vi "fu_gesamt.vi"(8 "Boolean":bool) -> (0 "Frequenz":dbl, 1 "Drehmoment":dbl format="%.2f", 2 "Leistung":dbl, 3 "Drehzahl":dbl, 11 "Scaled":dbl[](array[numeric]) format="%.2f")   [LabVIEW 2015]
uses:
  <vilib>/Instr/_visa.llb/VISA Configure Serial Port (Instr).vi
panel:
  out "return count":u32
  out "subarray":i8[](array[numeric])
  out "read buffer":string
  in  "VISA Refnum in":refnum<visa-resource-name>="COM1"
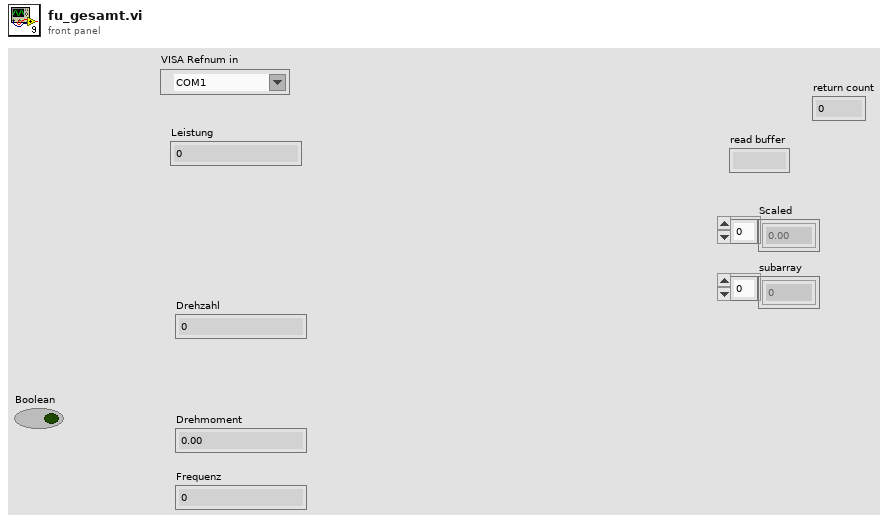
[diagram p1: front panel]
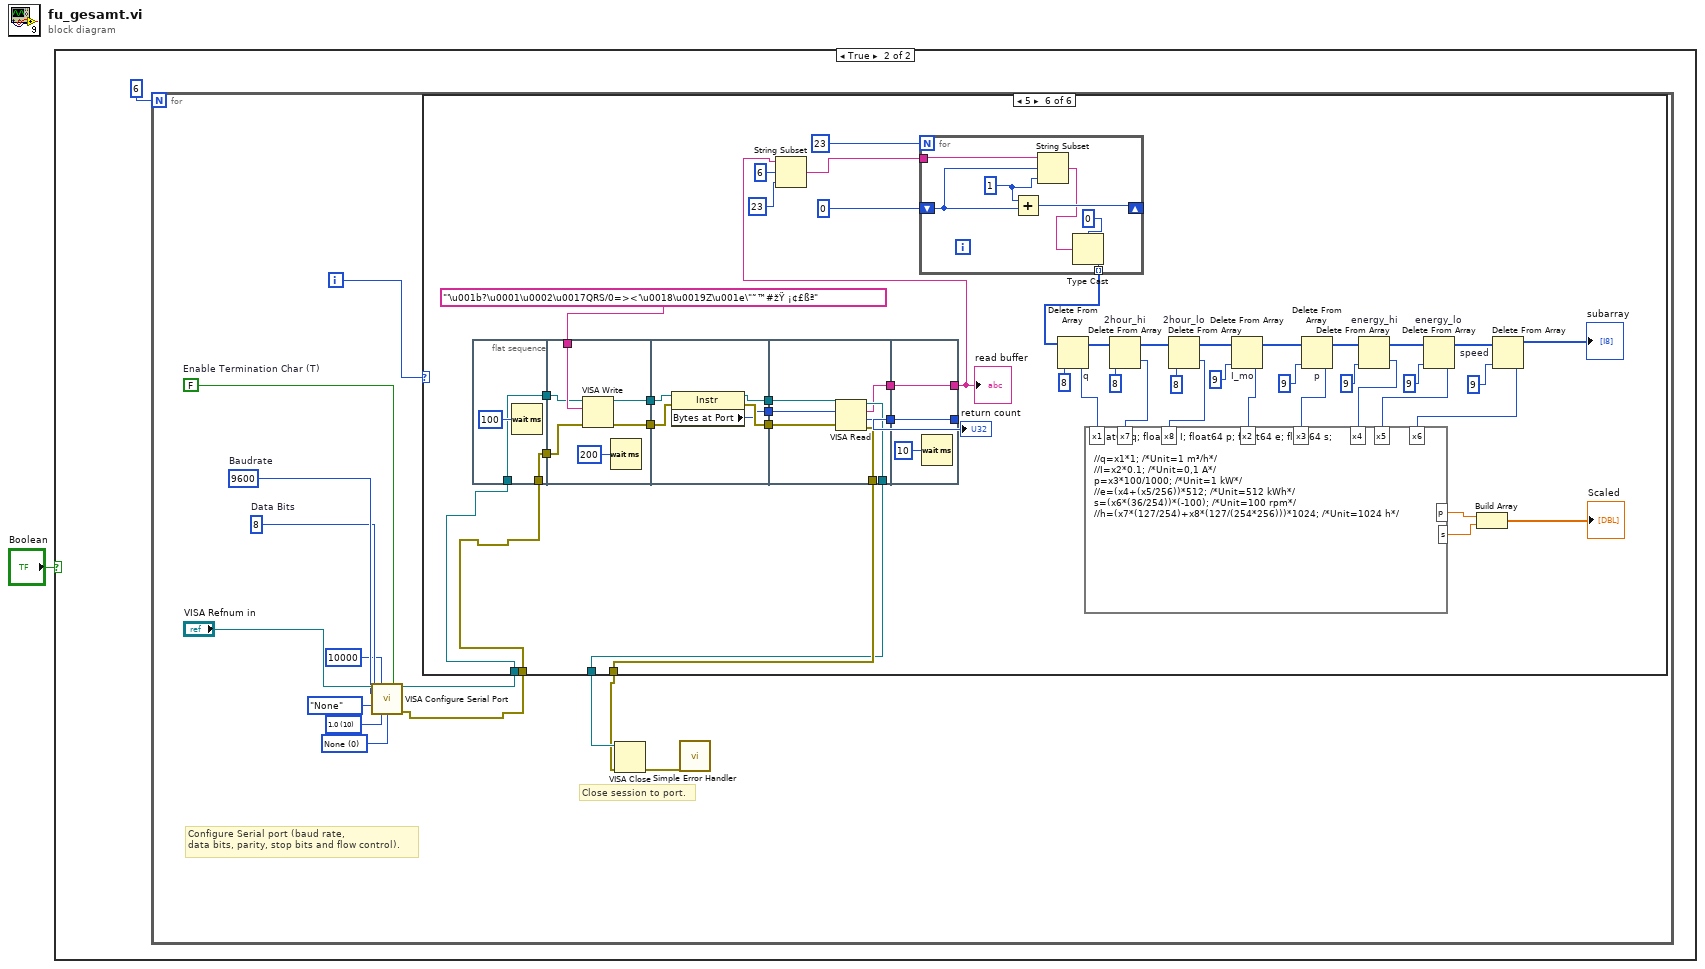
[diagram p0: block diagram]
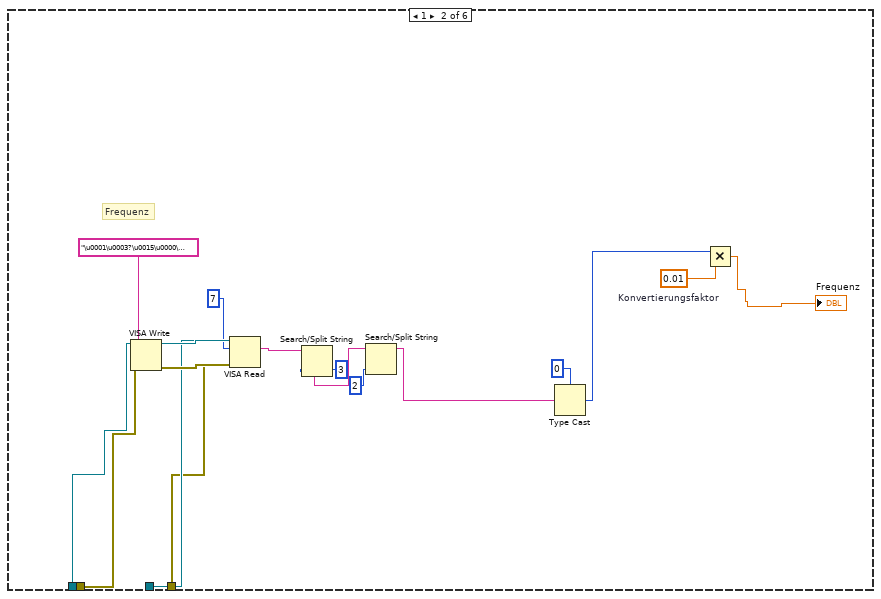
[diagram p4: hidden frame]
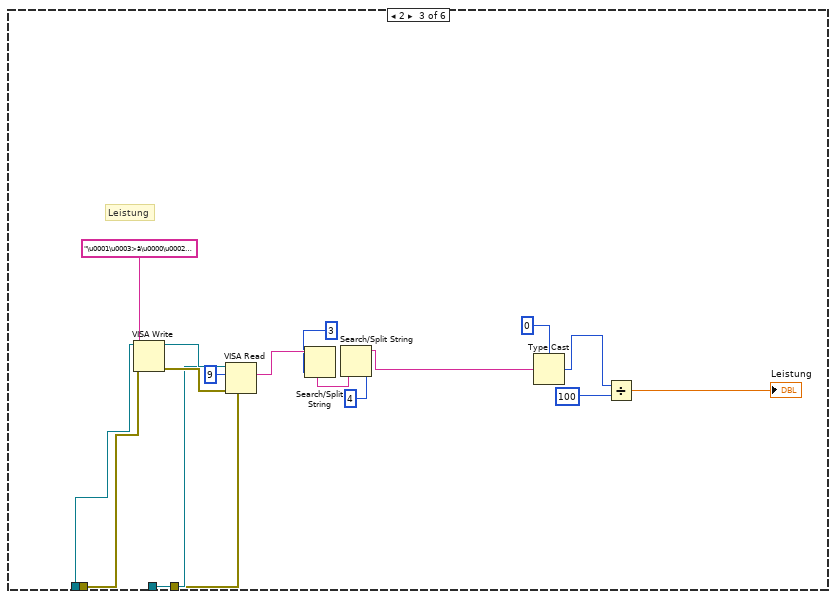
[diagram p5: hidden frame]
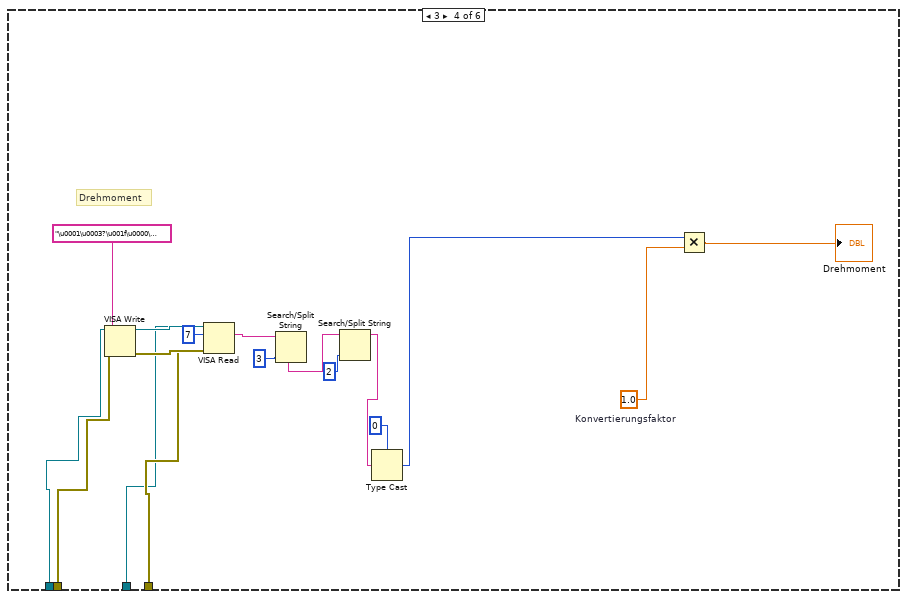
[diagram p6: hidden frame]
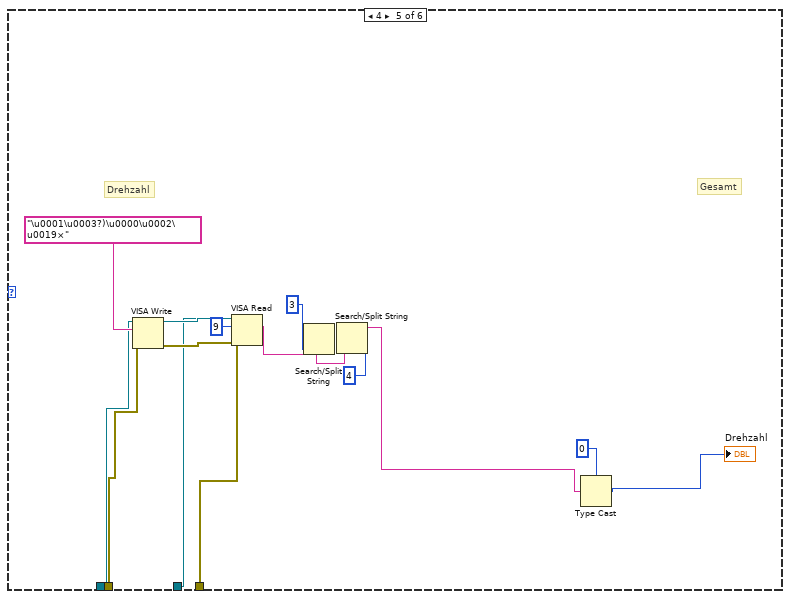
[diagram p7: hidden frame]
diagram:
  n1 = case shown="True" "Boolean" {
    frame False {
    }
    frame True {
      n2 = for {
        N: 6 -> [_]
        i -> [w7]
        w3 = u16 0 items=["None", "XON/XOFF", "RTS/CTS", "XON/XOFF & RTS/CTS", "DTR/DSR", "XON/XOFF & DTR/DSR"] ("flow control (0:none)")
        w4 = u16 10 items=["1.0"=10, "1.5"=15, "2.0"=20] ("stop bits (10: 1 bit)")
        w12 = u16 8  # Data Bits
        w13 = u32 9600  # Baudrate
        w15 = FALSE  # Enable Termination Char (T)
        # "Close session to port."
        # "Configure Serial port (baud rate,\ndata bits, parity, stop bits and flow control)."
        n3 = call-poly "VISA Configure Serial Port"("VISA resource name"="VISA Refnum in", "timeout (10sec)"=u32 10000, "Enable Termination\nChar (T)"=w15, "baud rate (9600)"=w13, "data bits (8)"=w12, "parity (0:none)"=enum16{"None", "Odd", "Even", "Mark", "Space"}."None", "stop bits (10: 1 bit)"=w4, "flow control (0:none)"=w3) -> ("VISA resource name out"=w8:refnum<visa-resource-name>, "error out"=w9:errorcluster)  [unwired: 6 in]
        n4 = case shown="5" w7 {
          tunnel: w8 -> [w18 w28 w45 w62 w78 w97]
          tunnel: [w18 w26 w43 w59 w76 w110] -> w11
          tunnel: [w17 w25 w42 w60 w75 w111] -> w10
          tunnel: w9 -> [w17 w27 w44 w61 w77 w96]
          frame 0, Default {
          }
          frame 1 {
            w24 = 0.01  # Konvertierungsfaktor
            # "Frequenz"
            n5 = VISA Write(VISA resource name=w28, write buffer="\u0001\u0003?\u0015\u0000\u0001™Ú", error in (no error)=w27) -> (VISA resource name out=w34:refnum<visa-resource-name>, error out=w35:errorcluster)  [unwired: 1 out]
            n6 = VISA Read(VISA resource name=w34, byte count=u32 7, error in (no error)=w35) -> (VISA resource name out=w26:refnum<visa-resource-name>, read buffer=w32:string, error out=w25:errorcluster)  [unwired: 1 out]
            n7 = Search/Split String(string=w32, offset (0)=3) -> (match + rest of string=w30:string)  [unwired: 1 in, 2 out]
            n8 = Search/Split String(string=w30, offset (0)=2) -> (substring before match=w23:string)  [unwired: 1 in, 2 out]
            n9 = Type Cast(type=i16 0, x=w23) -> (*(type *) &x=w22:i16)
            n10 = Multiply(x=w22, y=w24) -> (x*y=→"Frequenz":dbl)
          }
          frame 2 {
            # "Leistung"
            n11 = VISA Write(VISA resource name=w45, write buffer="\u0001\u0003>ã\u0000\u00028\u0015", error in (no error)=w44) -> (VISA resource name out=w51:refnum<visa-resource-name>, error out=w52:errorcluster)  [unwired: 1 out]
            n12 = VISA Read(VISA resource name=w51, byte count=u32 9, error in (no error)=w52) -> (VISA resource name out=w43:refnum<visa-resource-name>, read buffer=w49:string, error out=w42:errorcluster)  [unwired: 1 out]
            n13 = Search/Split String(string=w49, offset (0)=3) -> (match + rest of string=w47:string)  [unwired: 1 in, 2 out]
            n14 = Search/Split String(string=w47, offset (0)=4) -> (substring before match=w41:string)  [unwired: 1 in, 2 out]
            n15 = Type Cast(type=0, x=w41) -> (*(type *) &x=w40:i32)
            n16 = Divide(x=w40, y=100) -> (x/y=→"Leistung":dbl)
          }
          frame 3 {
            w54 = 1.0  # Konvertierungsfaktor
            # "Drehmoment"
            n17 = VISA Write(VISA resource name=w62, write buffer="\u0001\u0003?\u001f\u0000\u0001关", error in (no error)=w61) -> (VISA resource name out=w64:refnum<visa-resource-name>, error out=w63:errorcluster)  [unwired: 1 out]
            n18 = VISA Read(VISA resource name=w64, byte count=u32 7, error in (no error)=w63) -> (VISA resource name out=w59:refnum<visa-resource-name>, read buffer=w66:string, error out=w60:errorcluster)  [unwired: 1 out]
            n19 = Search/Split String(string=w66, offset (0)=3) -> (match + rest of string=w68:string)  [unwired: 1 in, 2 out]
            n20 = Search/Split String(string=w68, offset (0)=2) -> (substring before match=w58:string)  [unwired: 1 in, 2 out]
            n21 = Type Cast(type=i16 0, x=w58) -> (*(type *) &x=w57:i16)
            n22 = Multiply(x=w57, y=w54) -> (x*y=→"Drehmoment":dbl)
          }
          frame 4 {
            # "Gesamt"
            # "Drehzahl"
            n23 = VISA Write(VISA resource name=w78, write buffer="\u0001\u0003?)\u0000\u0002\u0019×", error in (no error)=w77) -> (VISA resource name out=w80:refnum<visa-resource-name>, error out=w79:errorcluster)  [unwired: 1 out]
            n24 = VISA Read(VISA resource name=w80, byte count=u32 9, error in (no error)=w79) -> (VISA resource name out=w76:refnum<visa-resource-name>, read buffer=w74:string, error out=w75:errorcluster)  [unwired: 1 out]
            n25 = Search/Split String(string=w74, offset (0)=3) -> (match + rest of string=w83:string)  [unwired: 1 in, 2 out]
            n26 = Search/Split String(string=w83, offset (0)=4) -> (substring before match=w73:string)  [unwired: 1 in, 2 out]
            n27 = Type Cast(type=0, x=w73) -> (*(type *) &x=→"Drehzahl":i32)
          }
          frame 5 {
            n28 = flat-sequence {
              tunnel: w97 -> [w135]
              tunnel: [w135] -> w99
              tunnel: w96 -> [w134]
              tunnel: [w134] -> w98
              tunnel: [w142] -> w106
              tunnel: [w141] -> w104
              tunnel: "'\u001b?\u0001\u0002\u0017QRS/0=><'\u0018\u0019Z\u001e\"˜™#žŸ ¡¢£ßª" -> [w140]
              tunnel: w99 -> [w138]
              tunnel: w98 -> [w137]
              tunnel: w106 -> [w147]
              tunnel: [w145] -> w105
              tunnel: w104 -> [w146]
              tunnel: [w144] -> w103
              tunnel: [w143] -> w100
              tunnel: w105 -> [w154]
              tunnel: w103 -> [w153]
              tunnel: [w152] -> w111
              tunnel: [w151] -> w110
              tunnel: [w150] -> w102
              tunnel: [w149] -> w101
              tunnel: w100 -> [w148]
              tunnel: [w156] -> w107
              tunnel: [w157] -> w108
              tunnel: w102 -> [w157]
              tunnel: w101 -> [w156]
              frame #0 {
                n29 = Wait (ms)(milliseconds to wait=u32 100) -> ()  [unwired: 1 out]
              }
              frame #1 {
                n30 = VISA Write(VISA resource name=w138, write buffer=w140, error in (no error)=w137) -> (VISA resource name out=w142:refnum<visa-resource-name>, error out=w141:errorcluster)  [unwired: 1 out]
                n31 = Wait (ms)(milliseconds to wait=u32 200) -> ()  [unwired: 1 out]
              }
              frame #2 {
                n32 = property class="Instr"(reference=w147, error in=w146) -> (reference out=w145:refnum<visa-resource-name>, error out=w144:errorcluster, "Bytes at Port"=w143:u32)
              }
              frame #3 {
                n33 = VISA Read(VISA resource name=w154, byte count=w148, error in (no error)=w153) -> (VISA resource name out=w151:refnum<visa-resource-name>, read buffer=w150:string, return count=w149:u32, error out=w152:errorcluster)
              }
              frame #4 {
                n34 = Wait (ms)(milliseconds to wait=u32 10) -> ()  [unwired: 1 out]
              }
            }
            n35 = String Subset(string=w108, offset (0)=6, length (rest)=23 ("length (rest)")) -> (substring=w92:string)
            n36 = for {
              N: 23 -> [_]
              tunnel: w92 -> [w164]
              shift-right: [w162] -> _
              shift-left: 0 -> [w161]
              tunnel: [w160] -> w112 mode=indexing
              w163 = 1
              n37 = Add(x=w163, y=w161) -> (x+y=w162:i32)
              n38 = String Subset(string=w164, offset (0)=w161, length (rest)=w163) -> (substring=w159:string)
              n39 = Type Cast(type=i8 0, x=w159) -> (*(type *) &x=w160:i8)
            }
            n40 = Delete From Array "q"(array=w112, index=8) -> (deleted portion=w119:i8, array with subset deleted=w91:i8[])  [unwired: 1 in]
            n41 = Delete From Array "2hour_hi"(array=w91, index=8) -> (deleted portion=w88:i8, array with subset deleted=w95:i8[])  [unwired: 1 in]
            n42 = Delete From Array "2hour_lo"(array=w95, index=8) -> (deleted portion=w87:i8, array with subset deleted=w90:i8[])  [unwired: 1 in]
            n43 = Delete From Array "I_mo"(array=w90, index=9) -> (deleted portion=w118:i8, array with subset deleted=w123:i8[])  [unwired: 1 in]
            n44 = Delete From Array "p"(array=w123, index=9) -> (deleted portion=w117:i8, array with subset deleted=w122:i8[])  [unwired: 1 in]
            n45 = Delete From Array "energy_hi"(array=w122, index=9) -> (deleted portion=w86:i8, array with subset deleted=w121:i8[])  [unwired: 1 in]
            n46 = Delete From Array "energy_lo"(array=w121, index=9) -> (deleted portion=w116:i8, array with subset deleted=w120:i8[])  [unwired: 1 in]
            n47 = Delete From Array "speed"(array=w120, index=9) -> (deleted portion=w115:i8, array with subset deleted=→"subarray":i8[])  [unwired: 1 in]
            n48 = formula code="float64 q; float64 I; float64 p; float64 e; float64 s;\n\n//q=x1*1; /*Unit=1 m³/h*/\n//I=x2*0.1; /*Unit=0,1 A*/\np=x3*100/1000; /*Unit=1 kW*/\n//e=(x4+(x5/256))*512; /*Unit=512 kWh*/\ns=(x6*(36/254))*(-100); /*Unit=100 rpm*/\n//h=(x7*(127/254)+x8*(127/(254*256)))*1024; /*Unit=1024 h*/"("x1"=w119, "x2"=w118, "x3"=w117, "x4"=w86, "x5"=w116, "x6"=w115, "x7"=w88, "x8"=w87) -> ("p"=w114:dbl, "s"=w113:dbl)
            n49 = Build Array(w114, w113) -> (→"Scaled":dbl[])
            "read buffer" <- w108
            "return count" <- w107
          }
        }
        n50 = VISA Close(VISA resource name=w11, error in (no error)=w10) -> (error out=w14:errorcluster)
        n51 = call <vilib>:"Simple Error Handler.vi"("error in (no error)"=w14) -> ()  [unwired: 4 in, 5 out]
      }
    }
  }
